vi "Write Boolean Text.vi"(8 "error in":errorcluster, 10 "Value":string[](array[string]), 11 "Boolean Reference in":refnum<vi>) -> (0 "error out":errorcluster, 3 "Boolean Reference out":refnum<vi>)   [LabVIEW 2020, in "G-Unicode.lvlib"]
uses:
  G-Unicode.lvlib
  <vilib>/Utility/miscctls.llb/LVSelectionTypeDef.ctl
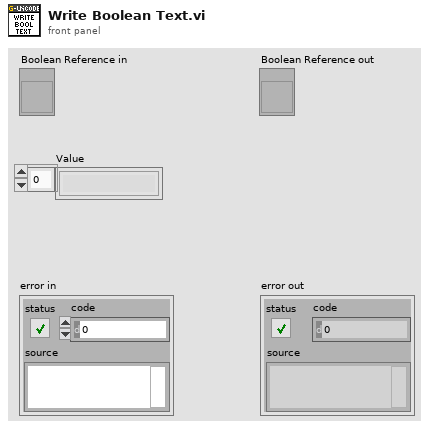
[diagram p1: front panel]
types:
  T1 = typedef "LVSelectionTypeDef.ctl" = cluster{"Selection Start":u32, "Selection End":u32}
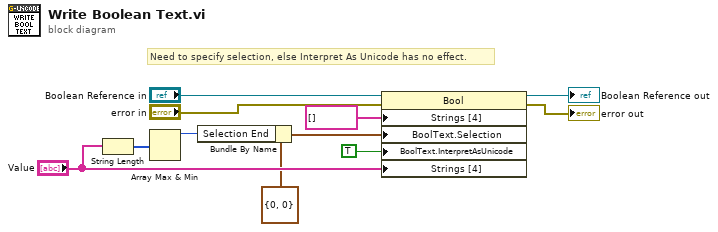
[diagram p0: block diagram]
diagram:
  # "Need to specify selection, else Interpret As Unicode has no effect."
  n1 = String Length(string="Value") -> (length=w4:i32[])
  n2 = Array Max & Min(array=w4) -> (max value=w2:i32)  [unwired: 3 out]
  n3 = Bundle By Name(cluster=T1 {"Selection Start"=0, "Selection End"=0} ("Boolean Text.Selection"), "Selection End"=w2) -> (w1:T1)
  n4 = property class="Bool"(reference="Boolean Reference in", error in="error in", "Strings [4]"=string[] [], "BoolText.Selection"=w1, "BoolText.InterpretAsUnicode"=TRUE ("Boolean Text.Interpret As Unicode"), "Strings [4]"="Value") -> (reference out=→"Boolean Reference out":refnum<vi>, error out=→"error out":errorcluster)
